vi "Agilent_34405A.vi"(0 "VISA resource name":refnum<visa-resource-name>="34405A", 1 "Enable Auto Range (T:Enable)":bool=TRUE, 5 "Op":T1(ring), 7 "DMM Mode (0: DC Volts)":u16(ring) format="%.0g" items=["DC Volts", "AC Volts", "DC Current", "AC Current", "2-Wire Resistance", "Frequency", "Temperature", "Capacitance", "Continuity", "Diode"], 9 "Init and config? (n)":bool, 11 "error in (no error)":errorcluster, 12 "Manual Range (10)":dbl=10.0) -> (3 "Return string":string, 4 "VISA resource name out":refnum<visa-resource-name>, 6 "First data item":dbl, 10 "Output Array":dbl[](array[numeric]) format="%.6e", 14 "First data item str":string, 15 "error out":errorcluster)   [LabVIEW 2013]
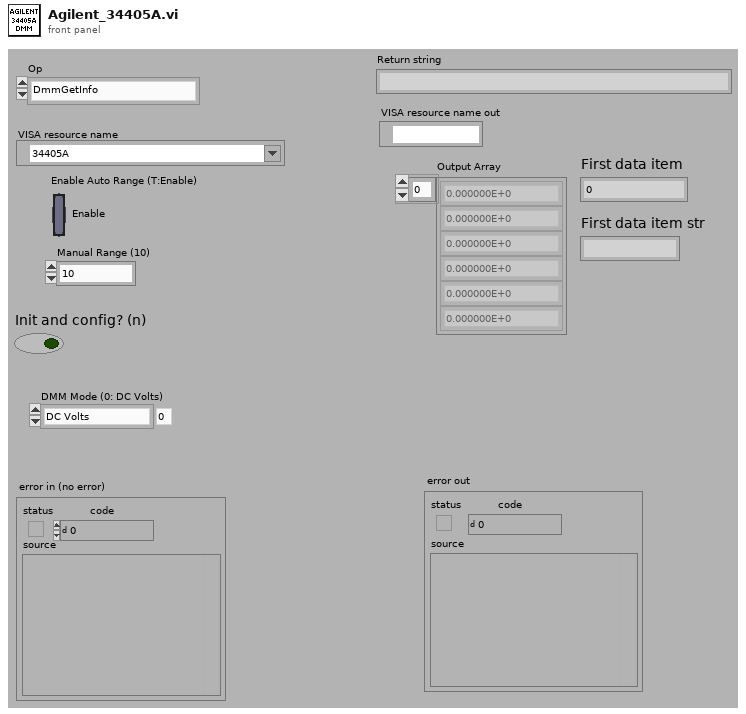
[diagram p1: front panel]
types:
  T1 = enum16{"DmmGetInfo", "DmmInit", "DmmOhms", "DmmDCvolts", "DmmACvolts", "DmmFreq", "DmmTemp", "DmmCap", "DmmAlarmHi", "DmmAlarmLow"}
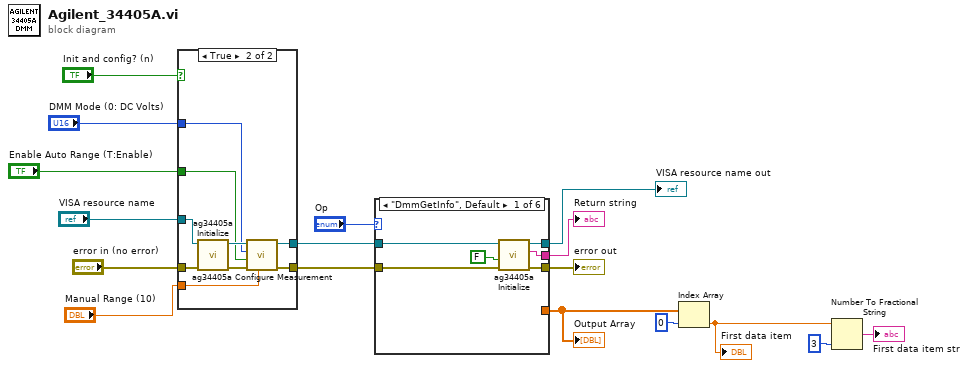
[diagram p0: block diagram]
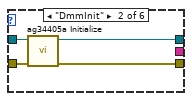
[diagram p3: hidden frame]
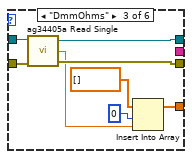
[diagram p4: hidden frame]
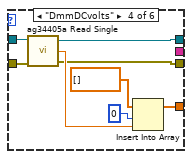
[diagram p5: hidden frame]
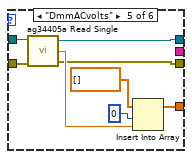
[diagram p6: hidden frame]
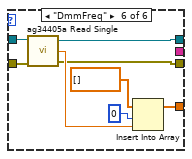
[diagram p7: hidden frame]
diagram:
  n1 = case shown="True" "Init and config? (n)" {
    tunnel: "error in (no error)" -> [w18 w26]
    tunnel: "VISA resource name" -> [w19 w25]
    tunnel: "Manual Range (10)" -> [_ w24]
    tunnel: "Enable Auto Range (T:Enable)" -> [_ w23]
    tunnel: [w19 w22] -> w4
    tunnel: [w18 w21] -> w3
    tunnel: "DMM Mode (0: DC Volts)" -> [_ w20]
    frame False {
    }
    frame True {
      n2 = call "ag34405a Initialize.vi"("error in (no error)"=w26, "VISA resource name"=w25) -> ("error out"=w28:errorcluster, "VISA resource name out"=w27:refnum<visa-resource-name>)  [unwired: 7 in, 1 out]
      n3 = call "ag34405a Configure Measurement.vi"("Manual Range (1)"=w24, "error in (no error)"=w28, "Enable Auto Range (T:Enable)"=w23, "Function (0: DC Volts)"=w20, "VISA resource name"=w27) -> ("error out"=w21:errorcluster, "VISA resource name out"=w22:refnum<visa-resource-name>)  [unwired: 5 in]
    }
  }
  n4 = case shown="\"DmmGetInfo\", Default" "Op" {
    tunnel: w4 -> [w34 w38 w43 w51 w56 w66]
    tunnel: w3 -> [w32 w37 w42 w50 w58 w65]
    tunnel: [w31 w36 w41 w49 w57 w64] -> w17
    tunnel: [_ _ w46 w48 w59 w67] -> w15
    tunnel: [w30 _ _ _ _ _] -> w16
    tunnel: [w29 w35 w39 w47 w55 w63] -> w10
    frame "DmmGetInfo", Default {
      n5 = call "ag34405a Initialize.vi"("error in (no error)"=w32, "Reset (True)"=FALSE, "VISA resource name"=w34) -> ("error out"=w31:errorcluster, "ID"=w30:string, "VISA resource name out"=w29:refnum<visa-resource-name>)  [unwired: 6 in]
    }
    frame "DmmInit" {
      n6 = call "ag34405a Initialize.vi"("error in (no error)"=w37, "VISA resource name"=w38) -> ("error out"=w36:errorcluster, "VISA resource name out"=w35:refnum<visa-resource-name>)  [unwired: 7 in, 1 out]
    }
    frame "DmmOhms" {
      n7 = call "ag34405a Read Single.vi"("VISA resource name"=w43, "error in (no error)"=w42) -> ("VISA resource name out"=w39:refnum<visa-resource-name>, "Measurement"=w40:dbl, "error out"=w41:errorcluster)  [unwired: 4 in]
      n8 = Insert Into Array(array=dbl[] [], index=0, new element=w40) -> (w46:dbl[])
    }
    frame "DmmDCvolts" {
      n9 = call "ag34405a Read Single.vi"("VISA resource name"=w51, "error in (no error)"=w50) -> ("VISA resource name out"=w47:refnum<visa-resource-name>, "Measurement"=w52:dbl, "error out"=w49:errorcluster)  [unwired: 4 in]
      n10 = Insert Into Array(array=dbl[] [], index=0, new element=w52) -> (w48:dbl[])
    }
    frame "DmmACvolts" {
      n11 = call "ag34405a Read Single.vi"("VISA resource name"=w56, "error in (no error)"=w58) -> ("VISA resource name out"=w55:refnum<visa-resource-name>, "Measurement"=w60:dbl, "error out"=w57:errorcluster)  [unwired: 4 in]
      n12 = Insert Into Array(array=dbl[] [], index=0, new element=w60) -> (w59:dbl[])
    }
    frame "DmmFreq" {
      n13 = call "ag34405a Read Single.vi"("VISA resource name"=w66, "error in (no error)"=w65) -> ("VISA resource name out"=w63:refnum<visa-resource-name>, "Measurement"=w68:dbl, "error out"=w64:errorcluster)  [unwired: 4 in]
      n14 = Insert Into Array(array=dbl[] [], index=0, new element=w68) -> (w67:dbl[])
    }
  }
  "error out" <- w17
  "Output Array" <- w15
  "Return string" <- w16
  "VISA resource name out" <- w10
  n15 = Index Array(array=w15, index=0) -> (element=w13:dbl)
  "First data item" <- w13
  n16 = Number To Fractional String(number=w13, precision (6)=i16 3) -> (F-format string=→"First data item str":string)  [unwired: 2 in]
